vi "uPolicy_TopicIsRelevant.vi"(8 "error in (no error)":errorcluster, 10 "Observed Topic (Lower Case)":string, 11 "uPolicy_All in":refnum<class "uPolicy.lvclass">) -> (0 "error out":errorcluster, 2 "Relevant?":bool, 3 "uPolicy_All out":refnum<class "uPolicy.lvclass">)   [LabVIEW 2021, in "uFramework.lvlib" / "uPolicy.lvclass"]
doc: "Dynamic dispatch method to allow the children to determine whether a topic is relevant to this subscription and provide the translated destination command where applicable.\n\nThe default behavior of the parent class is to pass any published event as is using the topic name as a destination command."
uses:
  uPolicy.lvclass
  uPolicy.lvclass/uPolicy.ctl
  Read uStringManipulation.vi
  uStringManipulation/uStringManipulation.lvclass
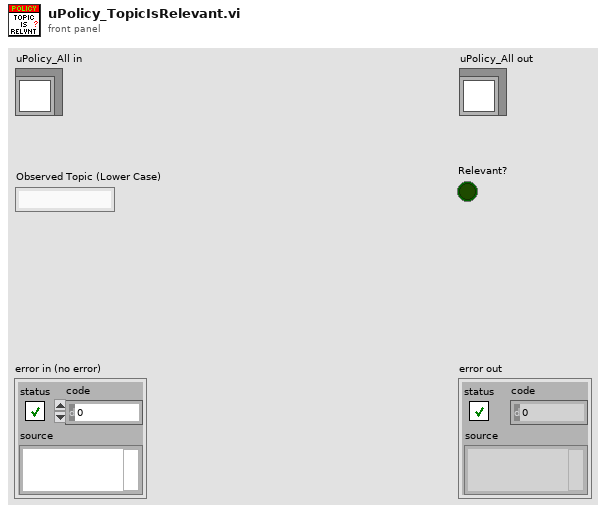
[diagram p1: front panel]
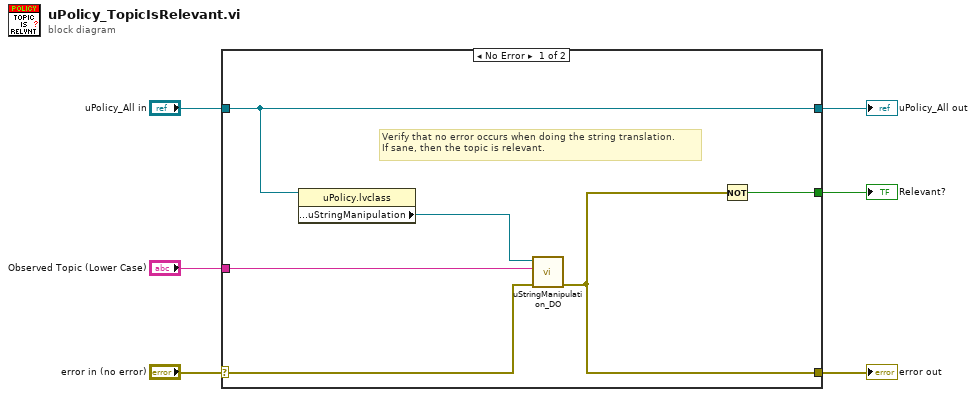
[diagram p0: block diagram]
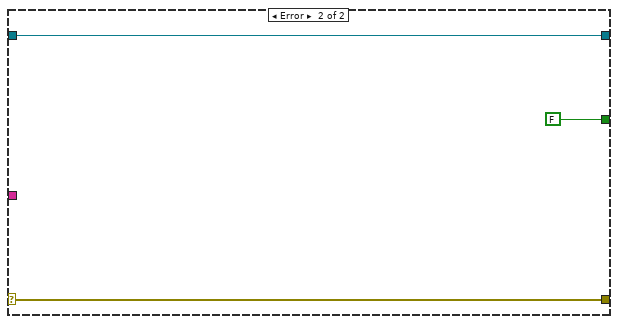
[diagram p2: hidden frame]
diagram:
  n1 = case shown="No Error" "error in (no error)" {
    selector: "error in (no error)" -> [w11 w15]
    tunnel: [w9 w15] -> w5
    tunnel: [w8 w14] -> w3
    tunnel: "uPolicy_All in" -> [w8 w14]
    tunnel: "Observed Topic (Lower Case)" -> [w12 _]
    tunnel: [w10 FALSE] -> w1
    frame No Error {
      # "Verify that no error occurs when doing the string translation.\nIf sane, then the topic is relevant."
      n2 = property class="uPolicy.lvclass"(reference=w8) -> ("PropertyNodes:uStringManipulation"=w7:refnum<class "uStringManipulation.lvclass">)  [unwired: 1 in, 2 out]
      n3 = call-dynamic "uStringManipulation_DO.vi"("error in (no error)"=w11, "String in"=w12, "uStringManipulation in"=w7) -> ("error out"=w9:errorcluster)  [unwired: 6 in, 2 out]
      n4 = Not(x=w9) -> (.not. x?=w10:bool)
    }
    frame Error {
    }
  }
  "error out" <- w5
  "uPolicy_All out" <- w3
  "Relevant?" <- w1
